vi "dsmmGeneratePlot.vi"(1 "Match":i32[](array[numeric]), 2 "Y":dbl[][](array[numeric]), 3 "X":dbl[][](array[numeric])) -> (0 "LV plot":cluster{dbl[], dbl[]}[](array[cluster]))   [LabVIEW 2017]
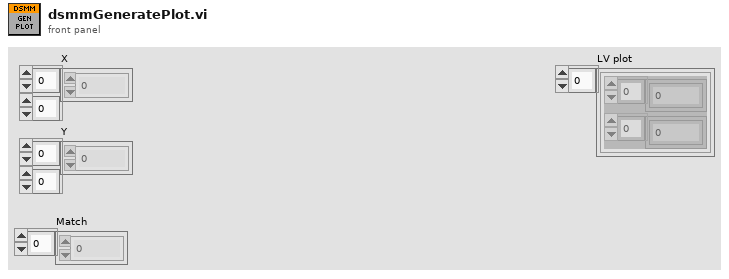
[diagram p1: front panel]
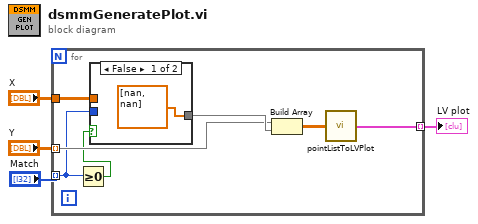
[diagram p0: block diagram]
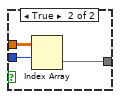
[diagram p2: hidden frame]
diagram:
  n1 = for {
    tunnel: "X" -> [w8]
    tunnel: "Y" -> [w7] mode=indexing
    tunnel: "Match" -> [w6] mode=indexing
    tunnel: [w9] -> w2 mode=indexing
    n2 = Greater Or Equal To 0?(x=w6) -> (x >= 0?=w5:bool)
    n3 = case shown="False" w5 {
      tunnel: w6 -> [_ w15]
      tunnel: [dbl[] [nan, nan] w14] -> w11
      tunnel: w8 -> [_ w13]
      frame False {
      }
      frame True {
        n4 = Index Array(array=w13, index (row)=w15) -> (element=w14:dbl[])  [unwired: 1 in]
      }
    }
    n5 = Build Array(w7, w11) -> (w10:dbl[][])
    n6 = call "pointListToLVPlot.vi"("XY[N,d]"=w10) -> ("LV plot"=w9:cluster{dbl[], dbl[]})
  }
  "LV plot" <- w2
